vi "Edit Poll.vi"(8 "error in (no error)":errorcluster, 11 "Node Ptr":u64 format="%.0x") -> (0 "error out":errorcluster)   [LabVIEW 2024, in "Diagnostics Addon System Explorer.lvlib"]
uses:
  Diagnostics Addon System Explorer.lvlib
  Types/FG.Action.ctl
  Types/Poll.LinkedNode.ctl
  <vilib>/NI VeriStand/Custom Device Tools/Custom Device Utility Library/Custom Device Utility Library.lvlib
  <vilib>/NI VeriStand/Custom Device API/Custom Device API.lvlib
panel:
  in  "Tag":string
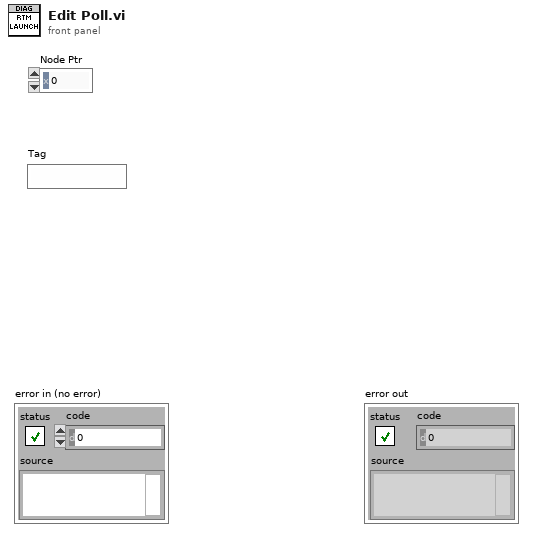
[diagram p1: front panel]
types:
  T1 = typedef "Diagnostics Addon System Explorer.lvlib/Poll.LinkedNode.ctl" = cluster{"Node ID":u64}
  T2 = typedef "Diagnostics Addon System Explorer.lvlib/FG.Action.ctl" = enum16{"Get", "Set"}
  T3 = typedef "Custom Device API.lvlib/Custom Device Item Info.ctl" = cluster{"Name":string, "Is Channel":bool, "GUID":string, "Is Waveform":bool}
  T4 = typedef "Custom Device API.lvlib/Custom Device Item Ref.ctl" = u64
  T5 = typedef "Diagnostics Addon System Explorer.lvlib/Poll.Settings.ctl" = cluster{"Input Channels":T1[], "Speed":T6}
  T6 = typedef "Diagnostics Addon Shared.lvlib/DPID.Rate.ctl" = enum16{"Slow", "Medium", "Fast"}
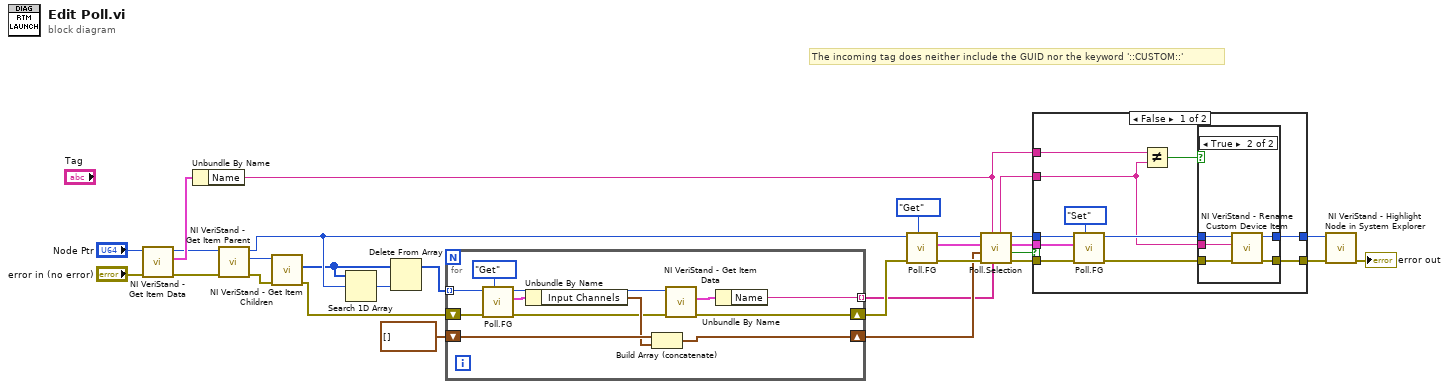
[diagram p0: block diagram]
diagram:
  # "The incoming tag does neither include the GUID nor the keyword '::CUSTOM::'"
  n1 = call <vilib>:"NI VeriStand - Get Item Data.vi"("error in (no error)"="error in (no error)", "Item Ref in"="Node Ptr") -> ("error out"=w5:errorcluster, "Item Info"=w9:T3, "Item Ref out"=w7:T4)  [unwired: 6 in, 1 out]
  n2 = Unbundle By Name(w9) -> ("Name"=w1:string)
  n3 = call <vilib>:"NI VeriStand - Get Item Parent.vi"("error in (no error)"=w5, "Item Ref in"=w7) -> ("error out"=w21:errorcluster, "Parent Ref"=w20:T4, "Item Ref out"=w19:T4)  [unwired: 6 in, 1 out]
  n4 = call <vilib>:"NI VeriStand - Get Item Children.vi"("error in (no error)"=w21, "Item Ref in"=w20) -> ("error out"=w15:errorcluster, "Child Refs"=w17:T4[])  [unwired: 6 in, 2 out]
  n5 = Search 1D Array(1D array=w17, element=w19) -> (index of element=w18:i32)  [unwired: 1 in]
  n6 = Delete From Array(array=w17, index=w18) -> (array with subset deleted=w16:T4[])  [unwired: 1 in, 1 out]
  n7 = for {
    tunnel: w16 -> [w39] mode=indexing
    shift-right: [w33] -> w13
    shift-left: w15 -> [w38]
    shift-right: [w35] -> w12
    shift-left: T1[] [] ("Input Channels") -> [w37]
    tunnel: [w30] -> w4 mode=indexing
    n8 = call "Poll.FG.vi"("Action"=FG.Action."Get", "error in"=w38, "Parent Ref"=w39) -> ("error out"=w34:errorcluster, "Selected Channels out"=w41:T5, "Parent Ref Out"=w32:T4)  [unwired: 6 in]
    n9 = Unbundle By Name(w41) -> ("Input Channels"=w36:T1[])
    n10 = Build Array (concatenate)(w37, w36) -> (w35:T1[])
    n11 = call <vilib>:"NI VeriStand - Get Item Data.vi"("error in (no error)"=w34, "Item Ref in"=w32) -> ("error out"=w33:errorcluster, "Item Info"=w31:T3)  [unwired: 6 in, 2 out]
    n12 = Unbundle By Name(w31) -> ("Name"=w30:string)
  }
  n13 = call "Poll.FG.vi"("Action"=FG.Action."Get", "error in"=w13, "Parent Ref"=w19) -> ("error out"=w26:errorcluster, "Selected Channels out"=w11:T5, "Parent Ref Out"=w27:T4)  [unwired: 6 in]
  n14 = call "Poll.Selection.vi"("Existing Names"=w4, "Name"=w1, "error in (no error)"=w26, "Already Used"=w12, "Selected Channels"=w11, "Node Ptr"=w27) -> ("error out"=w25:errorcluster, "Cancel out"=w3:bool, "Selected Channels"=w10:T5, "Node Ptr out"=w24:T4, "Name out"=w2:string)  [unwired: 1 in]
  n15 = case shown="False" w3 {
    tunnel: w25 -> [w51 w61]
    tunnel: w24 -> [w50 w60]
    tunnel: [w45 w61] -> w23
    tunnel: [w46 w60] -> w22
    tunnel: w10 -> [w49 _]
    tunnel: w2 -> [w44 _]
    tunnel: w1 -> [w43 _]
    frame False {
      n16 = call "Poll.FG.vi"("Action"=FG.Action."Set", "error in"=w51, "Selected Channels"=w49, "Parent Ref"=w50) -> ("error out"=w48:errorcluster, "Parent Ref Out"=w47:T4)  [unwired: 5 in, 1 out]
      n17 = Not Equal?(x=w43, y=w44) -> (x != y?=w42:bool)
      n18 = case shown="True" w42 {
        tunnel: w48 -> [w53 w59]
        tunnel: w47 -> [w54 w58]
        tunnel: [w54 w57] -> w46
        tunnel: [w53 w56] -> w45
        tunnel: w44 -> [_ w55]
        frame False {
        }
        frame True {
          n19 = call <vilib>:"NI VeriStand - Rename Custom Device Item.vi"("error in (no error)"=w59, "New Name"=w55, "Item Ref in"=w58) -> ("error out"=w56:errorcluster, "Item Ref out"=w57:T4)  [unwired: 6 in, 1 out]
        }
      }
    }
    frame True {
    }
  }
  n20 = call <vilib>:"NI VeriStand - Highlight Node in System Explorer.vi"("error in (no error)"=w23, "Item Ref in"=w22) -> ("error out"=→"error out":errorcluster)  [unwired: 8 in, 1 out]
